vi "TrapControllers1.vi"() -> ()   [LabVIEW 2016]
doc: "I. Description:\nThis example demonstrates how to continuously output a waveform using an internal sample clock. The automatic regeneration of data has been disabled, so new data has to be provided throughout the duration of the continuous Analog Output operation. This allows the generation of any arbitrary frequency as this VI computes new data for each iteration of the loop, maintaining phase continuity of the signal. The regeneration of data has also been adjusted so that the newest data is output as quickly as possible; thus reducing the lag between the changing of the data and the output of that data.\n\nII. Instructions for Running:\n1. Select the Physical Channel to correspond to where your signal is output on the DAQ device.\n2. Enter the Minimum and Maximum Voltage range.\n3. Specify the desired Sample Clock Rate of the output Waveform. Higher sample clock rates will produce a smoother waveform.\n4. Manually specify the Analog Output buffer size, in number of samples. A larger buffer would help non-regenerative operations avoid errors due to occasional high CPU load. \nNote: \nThe Analog Output buffer has to be at least as big as the amount of data being written to the board per iteration. The recommended buffer size would be at least twice the amount of data being written to the board per iteration.\n5. Enter the Waveform Information. See the documentation of the Basic Function Generator SubVI for information on each parameter.\n\nIII. Block Diagram Steps:\n1. Create an Analog Output Voltage channel.\n2. Configure the task to prohibit the automatic regeneration of data.\n2a. Set the transfer condition to Less than Full. Allows for more rapid updates of Output Buffer.\n3. Call the DAQmx (Sample Clock) VI to set the sample clock rate. Additionally, set the sample mode to Continuous.\n4. Read the actual sample clock rate (eventually coerced depending on the hardware used). \n5. Compute the desired waveform, using the buffer size and the actual update rate. This VI keeps track of the phase of the waveform to ensure that the generated signal is continuous.\n6. Write the waveform to the output buffer. \n7a. Call the Start VI. This is only needed when the loop is executed for the first time.\n7b. Do nothing.\n8. Loop continuously until user presses the Stop button. Every iteration computes and writes a new waveform to the buffer.\n9. Call the Clear Task VI to clear the Task.\n10. Use the popup dialog box to display an error or warning if any.\n\nIV. I/O Connections Overview:\nMake sure your signal output terminal matches the Physical Channel I/O Control. For further connection information, refer to your hardware reference manual."
panel:
  out "PZT_Caution":bool caption="Caution"
  in  "PZT_Time":u32=100 max=1000 step=1
  out "PZT_Z":i32
  out "PZT_Y":i32
  out "PZT_X":i32
  in  "PZT_Step":i32=1 min=0 max=1000 step=1
  in  "PZT_Center":bool
  in  "PZT_Z-":bool
  in  "PZT_Z+":bool
  in  "PZT_Y-":bool
  in  "PZT_Y+":bool
  in  "PZT_X+":bool
  in  "PZT_X-":bool
  out "PZT_ON":bool=TRUE
  in  "PZT_Start":bool
  out "PZT_Num":i32
  in  "PZT_Stop":bool
  in  "stop 5":bool
  out "Numeric 5":i32
  in  "OK Button 6":bool
  out "OK Button 5":bool
  out "OK Button 4":bool
  in  "stop 2":bool
  out "Numeric 4":i32
  in  "OK Button 2":bool
  in  "STOP":bool
  # "Stop all the sub controllers before STOP Program"
  # "Servo should be ON."
  # "Position (nm)"
  # "X"
  # "Y"
  # "Z"
  # "Trap Laser"
  # "Time (ms)"
  # "Step (nm)"
  # "Oscillation Mode"
  # "Manual Mode"
  # "PZT"
  # "LED"
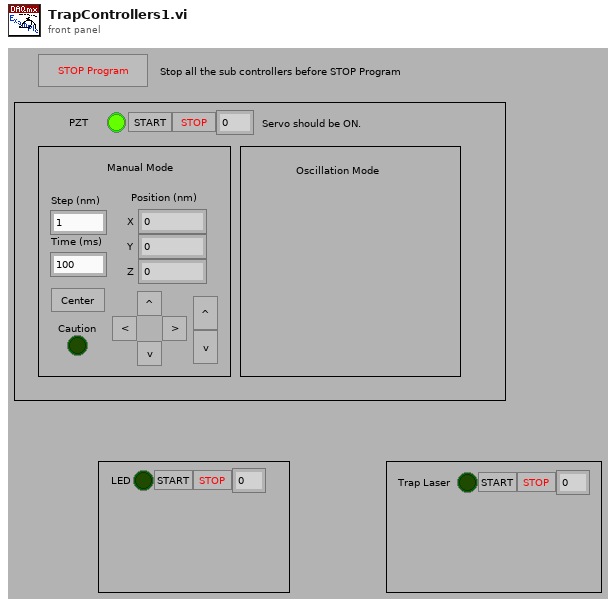
[diagram p1: front panel]
types:
  T1 = cluster{"PZT_X":i32, "PZT_Y":i32, "PZT_Z":i32, "PZT_Step":i32}
  T2 = typedef "eventvkey.ctl" = enum16{"ASCII", "Enter", "Return", "Shift", "Ctrl", "Alt", "Cmd", "Opt", "Caps", "NumLock", "Clear", "Break", "Up", "Down", "Left", "Right", "Insert", "Delete", "Home", "End", "PageUp", "PageDown", "Escape", "Help", "Pause", "ScrollLock", "F1", "F2", "F3", "F4", "F5", "F6", "F7", "F8", "F9", "F10", "F11", "F12", "F13", "F14", "F15", "F16", "F17", "F18", "F19", "F20", "F21", "F22", "F23", "F24", "Play", "VolumeUp", "VolumeDown", "Mute", "Two Byte Char"}
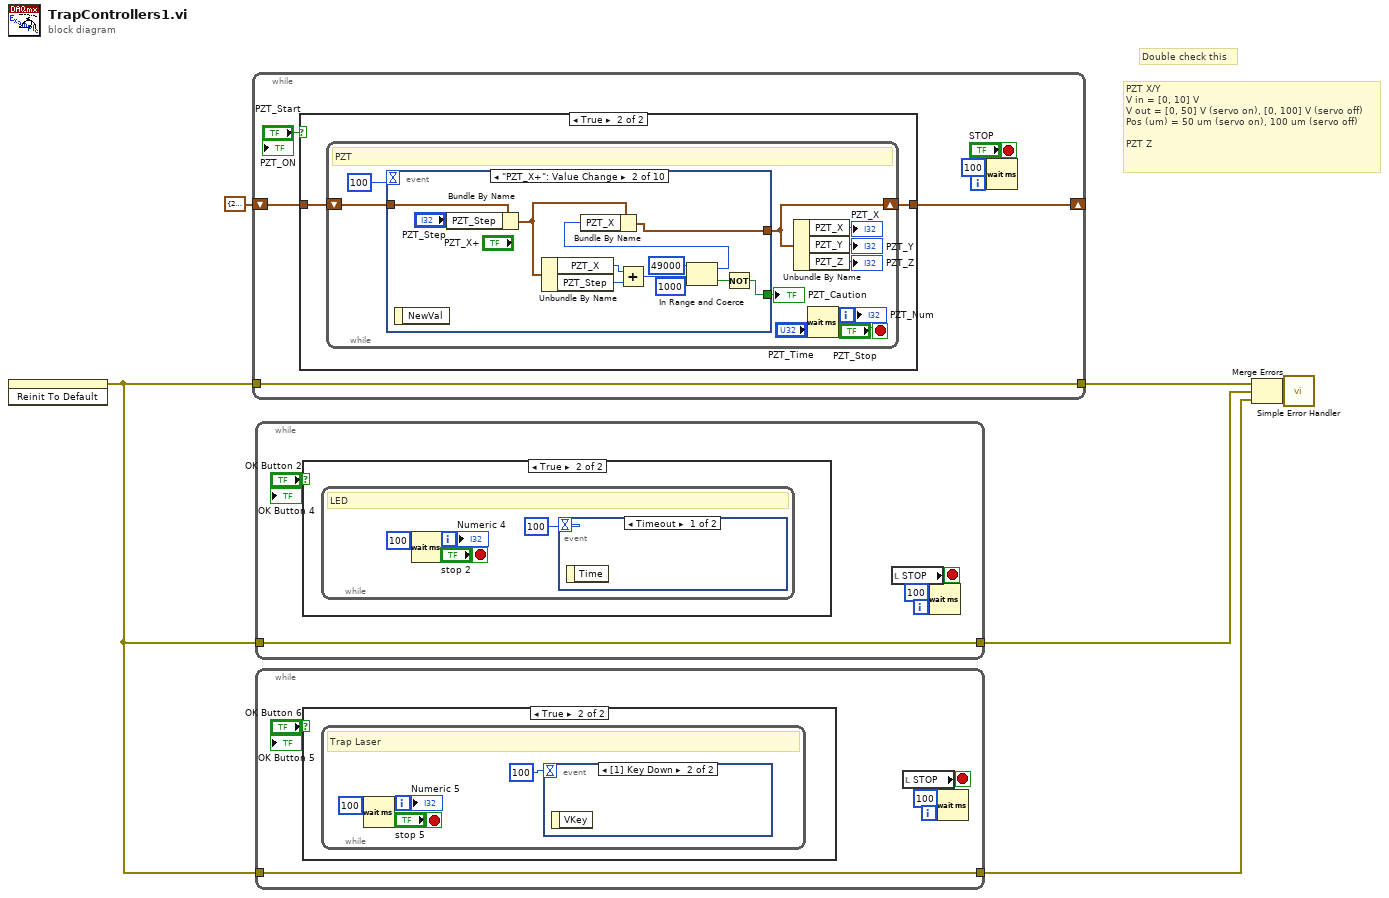
[diagram p0: block diagram]
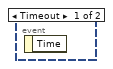
[diagram p3: hidden frame]
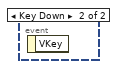
[diagram p5: hidden frame]
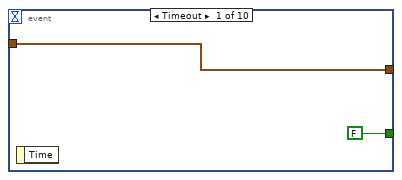
[diagram p7: hidden frame]
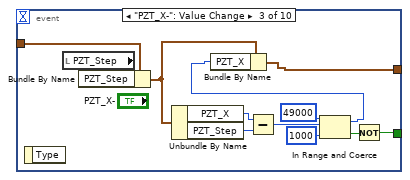
[diagram p8: hidden frame]
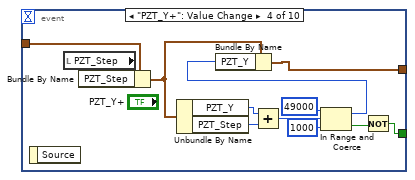
[diagram p9: hidden frame]
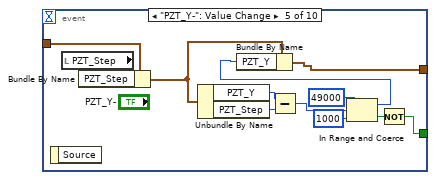
[diagram p10: hidden frame]
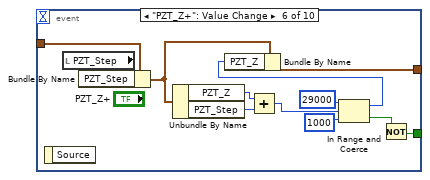
[diagram p11: hidden frame]
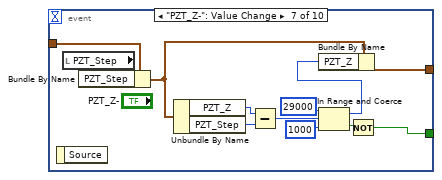
[diagram p12: hidden frame]
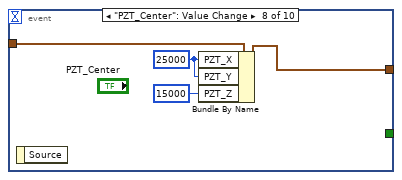
[diagram p13: hidden frame]
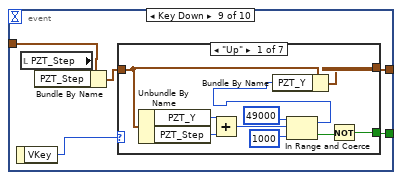
[diagram p14: hidden frame]
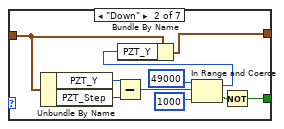
[diagram p15: hidden frame]
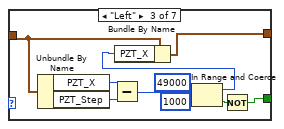
[diagram p16: hidden frame]
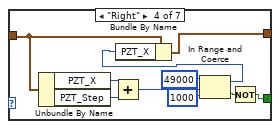
[diagram p17: hidden frame]
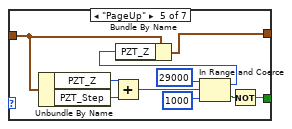
[diagram p18: hidden frame]
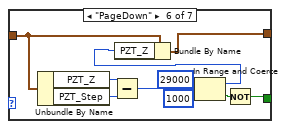
[diagram p19: hidden frame]
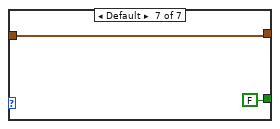
[diagram p20: hidden frame]
diagram:
  # "Double check this"
  # "PZT X/Y\nV in = [0, 10] V\nV out = [0, 50] V (servo on), [0, 100] V (servo off)\nPos (um) = 50 um (servo on), 100 um (servo off)\n\nPZT Z"
  n1 = invoke on="STOP" class="Bool (strict)" method="Reinit To Default"() -> (error out=w1:errorcluster)  [unwired: 3 in, 2 out]
  n2 = while {
    shift-right: [w10] -> _
    shift-left: T1 {"PZT_X"=25000, "PZT_Y"=25000, "PZT_Z"=15000, "PZT_Step"=10} ("output cluster") -> [w11]
    tunnel: [w9] -> w3
    tunnel: w1 -> [w9]
    stop <- "STOP" stop-if-true
    n3 = case shown="True" "PZT_Start" {
      tunnel: w11 -> [w13 w15]
      tunnel: [w13 w14] -> w10
      frame False {
      }
      frame True {
        n4 = while "Event Handle Loop" {
          shift-right: [w19] -> w14
          shift-left: w15 -> [w20]
          i -> [w25]
          stop <- "PZT_Stop" stop-if-true
          # "PZT"
          n5 = event shown="[1] \"PZT_X+\": Value Change" {
            selector: _ -> [_ _ _ _ _ _ _ _ _ _]
            dyn-events: _ -> [_ _ _ _ _ _ _ _ _ _]
            timeout: 100 -> [_ _ _ _ _ _ _ _ _ _]
            tunnel: w20 -> [w27 w35 w48 w60 w72 w84 w96 w103 w108 w176]
            tunnel: [w27 w36 w49 w61 w73 w85 w97 w102 w105 w173] -> w19
            tunnel: [FALSE w28 w42 w53 w67 w76 w88 _ w104 w172] -> w16
            event Timeout {
              n6 = event-data() -> ()  [unwired: 1 in, 1 out]
            }
            event "PZT_X+": Value Change {
              n7 = event-data() -> ()  [unwired: 1 in, 1 out]
              n8 = Bundle By Name(cluster=w35, "PZT_Step"="PZT_Step") -> (w34:T1)
              n9 = Unbundle By Name(w34) -> ("PZT_X"=w38:i32, "PZT_Step"=w37:i32)
              n10 = Add(x=w38, y=w37) -> (x+y=w31:i32)
              n11 = In Range and Coerce(upper limit=49000, x=w31, lower limit=1000) -> (coerced(x)=w30:i32, In Range?=w29:bool)
              n12 = Bundle By Name(cluster=w34, "PZT_X"=w30) -> (w36:T1)
              n13 = Not(x=w29) -> (.not. x?=w28:bool)
            }
            event "PZT_X-": Value Change {
              n14 = event-data() -> ()  [unwired: 1 in, 1 out]
              n15 = local read "PZT_Step"() -> (w46:i32)
              n16 = Bundle By Name(cluster=w48, "PZT_Step"=w46) -> (w47:T1)
              n17 = Unbundle By Name(w47) -> ("PZT_X"=w51:i32, "PZT_Step"=w50:i32)
              n18 = Subtract(x=w51, y=w50) -> (x-y=w43:i32)
              n19 = In Range and Coerce(upper limit=49000, x=w43, lower limit=1000) -> (coerced(x)=w41:i32, In Range?=w44:bool)
              n20 = Bundle By Name(cluster=w47, "PZT_X"=w41) -> (w49:T1)
              n21 = Not(x=w44) -> (.not. x?=w42:bool)
            }
            event "PZT_Y+": Value Change {
              n22 = event-data() -> ()  [unwired: 1 in, 1 out]
              n23 = local read "PZT_Step"() -> (w58:i32)
              n24 = Bundle By Name(cluster=w60, "PZT_Step"=w58) -> (w59:T1)
              n25 = Unbundle By Name(w59) -> ("PZT_Y"=w63:i32, "PZT_Step"=w62:i32)
              n26 = Add(x=w63, y=w62) -> (x+y=w55:i32)
              n27 = In Range and Coerce(upper limit=49000, x=w55, lower limit=1000) -> (coerced(x)=w54:i32, In Range?=w56:bool)
              n28 = Bundle By Name(cluster=w59, "PZT_Y"=w54) -> (w61:T1)
              n29 = Not(x=w56) -> (.not. x?=w53:bool)
            }
            event "PZT_Y-": Value Change {
              n30 = event-data() -> ()  [unwired: 1 in, 1 out]
              n31 = local read "PZT_Step"() -> (w70:i32)
              n32 = Bundle By Name(cluster=w72, "PZT_Step"=w70) -> (w71:T1)
              n33 = Unbundle By Name(w71) -> ("PZT_Y"=w75:i32, "PZT_Step"=w74:i32)
              n34 = Subtract(x=w75, y=w74) -> (x-y=w65:i32)
              n35 = In Range and Coerce(upper limit=49000, x=w65, lower limit=1000) -> (coerced(x)=w64:i32, In Range?=w68:bool)
              n36 = Bundle By Name(cluster=w71, "PZT_Y"=w64) -> (w73:T1)
              n37 = Not(x=w68) -> (.not. x?=w67:bool)
            }
            event "PZT_Z+": Value Change {
              n38 = event-data() -> ()  [unwired: 1 in, 1 out]
              n39 = local read "PZT_Step"() -> (w82:i32)
              n40 = Bundle By Name(cluster=w84, "PZT_Step"=w82) -> (w83:T1)
              n41 = Unbundle By Name(w83) -> ("PZT_Z"=w87:i32, "PZT_Step"=w86:i32)
              n42 = Add(x=w87, y=w86) -> (x+y=w79:i32)
              n43 = In Range and Coerce(upper limit=29000, x=w79, lower limit=1000) -> (coerced(x)=w77:i32, In Range?=w80:bool)
              n44 = Bundle By Name(cluster=w83, "PZT_Z"=w77) -> (w85:T1)
              n45 = Not(x=w80) -> (.not. x?=w76:bool)
            }
            event "PZT_Z-": Value Change {
              n46 = event-data() -> ()  [unwired: 1 in, 1 out]
              n47 = local read "PZT_Step"() -> (w94:i32)
              n48 = Bundle By Name(cluster=w96, "PZT_Step"=w94) -> (w95:T1)
              n49 = Unbundle By Name(w95) -> ("PZT_Z"=w99:i32, "PZT_Step"=w98:i32)
              n50 = Subtract(x=w99, y=w98) -> (x-y=w91:i32)
              n51 = In Range and Coerce(upper limit=29000, x=w91, lower limit=1000) -> (coerced(x)=w89:i32, In Range?=w92:bool)
              n52 = Bundle By Name(cluster=w95, "PZT_Z"=w89) -> (w97:T1)
              n53 = Not(x=w92) -> (.not. x?=w88:bool)
            }
            event "PZT_Center": Value Change {
              w101 = 25000 ("PZT_X")
              n54 = event-data() -> ()  [unwired: 1 in, 1 out]
              n55 = Bundle By Name(cluster=w103, "PZT_X"=w101, "PZT_Y"=w101, "PZT_Z"=15000) -> (w102:T1)
            }
            event Key Down {
              n56 = event-data() -> ("VKey"=w109:T2)  [unwired: 1 in]
              n57 = local read "PZT_Step"() -> (w107:i32)
              n58 = Bundle By Name(cluster=w108, "PZT_Step"=w107) -> (w106:T1)
              n59 = case shown="\"Up\"" w109 {
                tunnel: w106 -> [w117 w127 w137 w147 w157 w167 w171]
                tunnel: [w116 w126 w136 w146 w156 w166 w171] -> w105
                tunnel: [w111 w122 w132 w142 w152 w162 FALSE] -> w104
                frame "Up" {
                  n60 = Unbundle By Name(w117) -> ("PZT_Y"=w119:i32, "PZT_Step"=w118:i32)
                  n61 = Add(x=w119, y=w118) -> (x+y=w113:i32)
                  n62 = In Range and Coerce(upper limit=49000, x=w113, lower limit=1000) -> (coerced(x)=w110:i32, In Range?=w114:bool)
                  n63 = Bundle By Name(cluster=w117, "PZT_Y"=w110) -> (w116:T1)
                  n64 = Not(x=w114) -> (.not. x?=w111:bool)
                }
                frame "Down" {
                  n65 = Unbundle By Name(w127) -> ("PZT_Y"=w129:i32, "PZT_Step"=w128:i32)
                  n66 = Subtract(x=w129, y=w128) -> (x-y=w121:i32)
                  n67 = In Range and Coerce(upper limit=49000, x=w121, lower limit=1000) -> (coerced(x)=w120:i32, In Range?=w124:bool)
                  n68 = Bundle By Name(cluster=w127, "PZT_Y"=w120) -> (w126:T1)
                  n69 = Not(x=w124) -> (.not. x?=w122:bool)
                }
                frame "Left" {
                  n70 = Unbundle By Name(w137) -> ("PZT_X"=w139:i32, "PZT_Step"=w138:i32)
                  n71 = Subtract(x=w139, y=w138) -> (x-y=w131:i32)
                  n72 = In Range and Coerce(upper limit=49000, x=w131, lower limit=1000) -> (coerced(x)=w130:i32, In Range?=w134:bool)
                  n73 = Bundle By Name(cluster=w137, "PZT_X"=w130) -> (w136:T1)
                  n74 = Not(x=w134) -> (.not. x?=w132:bool)
                }
                frame "Right" {
                  n75 = Unbundle By Name(w147) -> ("PZT_X"=w149:i32, "PZT_Step"=w148:i32)
                  n76 = Add(x=w149, y=w148) -> (x+y=w141:i32)
                  n77 = In Range and Coerce(upper limit=49000, x=w141, lower limit=1000) -> (coerced(x)=w140:i32, In Range?=w144:bool)
                  n78 = Bundle By Name(cluster=w147, "PZT_X"=w140) -> (w146:T1)
                  n79 = Not(x=w144) -> (.not. x?=w142:bool)
                }
                frame "PageUp" {
                  n80 = Unbundle By Name(w157) -> ("PZT_Z"=w159:i32, "PZT_Step"=w158:i32)
                  n81 = Add(x=w159, y=w158) -> (x+y=w151:i32)
                  n82 = In Range and Coerce(upper limit=29000, x=w151, lower limit=1000) -> (coerced(x)=w150:i32, In Range?=w154:bool)
                  n83 = Bundle By Name(cluster=w157, "PZT_Z"=w150) -> (w156:T1)
                  n84 = Not(x=w154) -> (.not. x?=w152:bool)
                }
                frame "PageDown" {
                  n85 = Unbundle By Name(w167) -> ("PZT_Z"=w169:i32, "PZT_Step"=w168:i32)
                  n86 = Subtract(x=w169, y=w168) -> (x-y=w161:i32)
                  n87 = In Range and Coerce(upper limit=29000, x=w161, lower limit=1000) -> (coerced(x)=w160:i32, In Range?=w164:bool)
                  n88 = Bundle By Name(cluster=w167, "PZT_Z"=w160) -> (w166:T1)
                  n89 = Not(x=w164) -> (.not. x?=w162:bool)
                }
                frame Default {
                }
              }
            }
            event Key Repeat {
              n90 = event-data() -> ("VKey"=w177:T2)  [unwired: 1 in]
              n91 = local read "PZT_Step"() -> (w175:i32)
              n92 = Bundle By Name(cluster=w176, "PZT_Step"=w175) -> (w174:T1)
              n93 = case shown="Default" w177 {
                tunnel: w174 -> [w185 w195 w205 w215 w225 w235 w239]
                tunnel: [w184 w194 w204 w214 w224 w234 w239] -> w173
                tunnel: [w178 w188 w198 w208 w218 w228 FALSE] -> w172
                frame "Up" {
                  n94 = Unbundle By Name(w185) -> ("PZT_Y"=w187:i32, "PZT_Step"=w186:i32)
                  n95 = Add(x=w187, y=w186) -> (x+y=w183:i32)
                  n96 = In Range and Coerce(upper limit=49000, x=w183, lower limit=1000) -> (coerced(x)=w182:i32, In Range?=w179:bool)
                  n97 = Bundle By Name(cluster=w185, "PZT_Y"=w182) -> (w184:T1)
                  n98 = Not(x=w179) -> (.not. x?=w178:bool)
                }
                frame "Down" {
                  n99 = Unbundle By Name(w195) -> ("PZT_Y"=w197:i32, "PZT_Step"=w196:i32)
                  n100 = Subtract(x=w197, y=w196) -> (x-y=w193:i32)
                  n101 = In Range and Coerce(upper limit=49000, x=w193, lower limit=1000) -> (coerced(x)=w190:i32, In Range?=w189:bool)
                  n102 = Bundle By Name(cluster=w195, "PZT_Y"=w190) -> (w194:T1)
                  n103 = Not(x=w189) -> (.not. x?=w188:bool)
                }
                frame "Left" {
                  n104 = Unbundle By Name(w205) -> ("PZT_X"=w207:i32, "PZT_Step"=w206:i32)
                  n105 = Subtract(x=w207, y=w206) -> (x-y=w203:i32)
                  n106 = In Range and Coerce(upper limit=49000, x=w203, lower limit=1000) -> (coerced(x)=w200:i32, In Range?=w199:bool)
                  n107 = Bundle By Name(cluster=w205, "PZT_X"=w200) -> (w204:T1)
                  n108 = Not(x=w199) -> (.not. x?=w198:bool)
                }
                frame "Right" {
                  n109 = Unbundle By Name(w215) -> ("PZT_X"=w217:i32, "PZT_Step"=w216:i32)
                  n110 = Add(x=w217, y=w216) -> (x+y=w213:i32)
                  n111 = In Range and Coerce(upper limit=49000, x=w213, lower limit=1000) -> (coerced(x)=w210:i32, In Range?=w209:bool)
                  n112 = Bundle By Name(cluster=w215, "PZT_X"=w210) -> (w214:T1)
                  n113 = Not(x=w209) -> (.not. x?=w208:bool)
                }
                frame "PageUp" {
                  n114 = Unbundle By Name(w225) -> ("PZT_Z"=w227:i32, "PZT_Step"=w226:i32)
                  n115 = Add(x=w227, y=w226) -> (x+y=w223:i32)
                  n116 = In Range and Coerce(upper limit=29000, x=w223, lower limit=1000) -> (coerced(x)=w220:i32, In Range?=w219:bool)
                  n117 = Bundle By Name(cluster=w225, "PZT_Z"=w220) -> (w224:T1)
                  n118 = Not(x=w219) -> (.not. x?=w218:bool)
                }
                frame "PageDown" {
                  n119 = Unbundle By Name(w235) -> ("PZT_Z"=w237:i32, "PZT_Step"=w236:i32)
                  n120 = Subtract(x=w237, y=w236) -> (x-y=w233:i32)
                  n121 = In Range and Coerce(upper limit=29000, x=w233, lower limit=1000) -> (coerced(x)=w230:i32, In Range?=w229:bool)
                  n122 = Bundle By Name(cluster=w235, "PZT_Z"=w230) -> (w234:T1)
                  n123 = Not(x=w229) -> (.not. x?=w228:bool)
                }
                frame Default {
                }
              }
            }
          }
          "PZT_Caution" <- w16
          n124 = Unbundle By Name(w19) -> ("PZT_X"=→"PZT_X":i32, "PZT_Y"=→"PZT_Y":i32, "PZT_Z"=→"PZT_Z":i32)
          n125 = Wait (ms)(milliseconds to wait="PZT_Time") -> ()  [unwired: 1 out]
          "PZT_Num" <- w25
        }
      }
    }
    n126 = Wait (ms)(milliseconds to wait=u32 100) -> ()  [unwired: 1 out]
    "PZT_ON" <- "PZT_Start"
  }
  n127 = while {
    tunnel: w1 -> [w241]
    tunnel: [w241] -> w5
    stop <- w242 stop-if-true
    n128 = case shown="True" "OK Button 2" {
      frame False {
      }
      frame True {
        n129 = while "Event Handle Loop" {
          i -> [w246]
          stop <- "stop 2" stop-if-true
          # "LED"
          n130 = Wait (ms)(milliseconds to wait=u32 100) -> ()  [unwired: 1 out]
          n131 = event shown="[0] Timeout" {
            selector: _ -> [_ _]
            dyn-events: _ -> [_ _]
            timeout: 100 -> [_ _]
            event Timeout {
              n132 = event-data() -> ()  [unwired: 1 in, 1 out]
            }
            event Key Down {
              n133 = event-data() -> ()  [unwired: 1 in, 1 out]
            }
          }
          "Numeric 4" <- w246
        }
      }
    }
    n134 = local read "STOP"() -> (w242:bool)
    n135 = Wait (ms)(milliseconds to wait=u32 100) -> ()  [unwired: 1 out]
    "OK Button 4" <- "OK Button 2"
  }
  n136 = while {
    tunnel: w1 -> [w249]
    tunnel: [w249] -> w4
    stop <- w250 stop-if-true
    n137 = case shown="True" "OK Button 6" {
      frame False {
      }
      frame True {
        n138 = while "Event Handle Loop" {
          i -> [w253]
          stop <- "stop 5" stop-if-true
          # "Trap Laser"
          n139 = Wait (ms)(milliseconds to wait=u32 100) -> ()  [unwired: 1 out]
          n140 = event shown="[1] Key Down" {
            selector: _ -> [_ _]
            dyn-events: _ -> [_ _]
            timeout: 100 -> [_ _]
            event Timeout {
              n141 = event-data() -> ()  [unwired: 1 in, 1 out]
            }
            event Key Down {
              n142 = event-data() -> ()  [unwired: 1 in, 1 out]
            }
          }
          "Numeric 5" <- w253
        }
      }
    }
    n143 = local read "STOP"() -> (w250:bool)
    n144 = Wait (ms)(milliseconds to wait=u32 100) -> ()  [unwired: 1 out]
    "OK Button 5" <- "OK Button 6"
  }
  n145 = Merge Errors(w3, w5, w4) -> (w6:errorcluster)
  n146 = call <vilib>:"Simple Error Handler.vi"("error in (no error)"=w6) -> ()  [unwired: 4 in, 5 out]
